vi "GetDLLPath.vi"(9 "DllName_32bit":string, 11 "DllName_64bit":string) -> (2 "file exists?":bool, 3 "DLLPath":path)   [LabVIEW 2010]
uses:
  <vilib>/Utility/sysdir.llb/System Directory Type.ctl
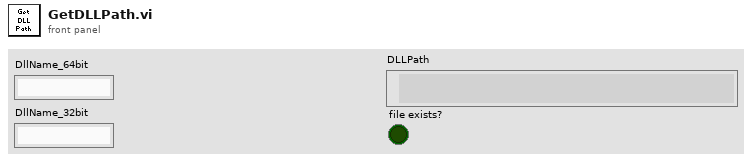
[diagram p1: front panel]
types:
  T1 = typedef "System Directory Type.ctl" = i32
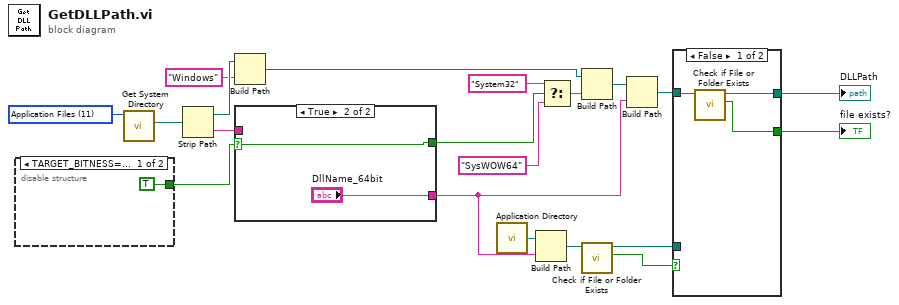
[diagram p0: block diagram]
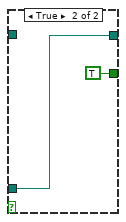
[diagram p2: hidden frame]
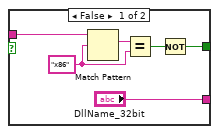
[diagram p3: hidden frame]
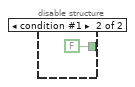
[diagram p4: hidden frame]
diagram:
  w20 = T1 11 items=["User Home"=0, "User Desktop"=1, "User Documents"=2, "User Application Data"=3, "User Preferences"=4, "User Temporary"=5, "Public Documents"=6, "Public Application Data"=7, "Public Preferences"=8, "Public Cache"=13, "System Core Libraries"=9, "System Installed Libraries"=10, "Application Files"=11, "Boot Volume Root"=12] ("system directory type")
  n1 = disable-structure shown="TARGET_BITNESS==64, Default" {
    disable-tunnel: [TRUE FALSE] -> w12
    frame condition #0 (active) {
    }
    frame condition #1 {
    }
  }
  n2 = call <vilib>:"Get System Directory.vi"("system directory type"=w20) -> ("system directory"=w19:path)  [unwired: 10 in]
  n3 = Strip Path(path=w19) -> (stripped path=w18:path, name=w10:string)
  n4 = Build Path(base path=w18, name or relative path="Windows") -> (appended path=w16:path)
  n5 = case shown="True" w12 {
    selector: w12 -> [_ w30]
    tunnel: [w24 w30] -> w11
    tunnel: w10 -> [w28 _]
    tunnel: ["DllName_32bit" "DllName_64bit"] -> w7
    frame False {
      w27 = "x86" ("regular expression")
      n6 = Match Pattern(string=w28, regular expression=w27) -> (match substring=w26:string)  [unwired: 1 in, 3 out]
      n7 = Equal?(x=w26, y=w27) -> (x = y?=w25:bool)
      n8 = Not(x=w25) -> (.not. x?=w24:bool)
    }
    frame True {
    }
  }
  n9 = call <vilib>:"Application Directory.vi"() -> ("Application Directory"=w8:path)
  n10 = Build Path(base path=w8, name or relative path=w7) -> (appended path=w6:path)
  n11 = Select(t="System32" ("name or relative path"), s=w11, f="SysWOW64" ("name or relative path")) -> (s? t:f=w14:string)
  n12 = Build Path(base path=w16, name or relative path=w14) -> (appended path=w9:path)
  n13 = call <vilib>:"Check if File or Folder Exists.vi"("path"=w6) -> ("file or folder exists?"=w5:bool, "dup path"=w1:path)  [unwired: 8 in, 1 out]
  n14 = Build Path(base path=w9, name or relative path=w7) -> (appended path=w4:path)
  n15 = case shown="False" w5 {
    tunnel: w4 -> [w33 _]
    tunnel: [w32 TRUE ("file or folder exists?")] -> w3
    tunnel: [w31 w35] -> w2
    tunnel: w1 -> [_ w35]
    frame False {
      n16 = call <vilib>:"Check if File or Folder Exists.vi"("path"=w33) -> ("file or folder exists?"=w32:bool, "dup path"=w31:path)  [unwired: 8 in, 1 out]
    }
    frame True {
    }
  }
  "DLLPath" <- w2
  "file exists?" <- w3
